vi "data_analysis main_correct.vi"() -> ()   [LabVIEW 2017]
uses:
  <vilib>/Analysis/baseanly.llb/Mean (DBL).vi
  <vilib>/Waveform/WDTFileIO.llb/Export Waveforms To Spreadsheet File (1D).vi
  <vilib>/Utility/file.llb/Read From Spreadsheet File (DBL).vi
  <vilib>/Analysis/NI_AALBase.lvlib
panel:
  in  "停止":bool
  out "Zmag trajectory":waveform(dbl) caption="元素"
  out "Ext.":dbl
  out "Z pos":waveform(dbl)(graph)
  out "Zmag pos":waveform(dbl)(graph)
  out "data name":string
  out "cursor pos":dbl
  out "cursor length":dbl
  out "zmag cursor pos":dbl
  out "zmag cursor length":dbl
  out "current bead":string
  in  "graphs":enum32{"raw data", "force calculation"}(tab)
  out "XY图":cluster{dbl[], dbl[]}(graph)
  in  "ref NO.":i32 min=0
  in  "remove drift":bool
  in  "sample rate":dbl=100.0
  in  "zero point offset":bool
  out "x_0":dbl caption="X0" format="%0.2f"
  out "y_0":dbl caption="Y0" format="%0.2f"
  out "z_0":dbl caption="Z0" format="%0.2f"
  in  "file save path":path
  in  "数据另存为":bool
  in  "data type":enum16{"tdms", "gr", "excel"}(ring)
  out "保存完成？":bool
  in  "file path":path
  in  "load data":bool
  in  "data info":i32(listbox)
  in  "bead NO.":i32 min=0
  in  "trajectory":i32 min=0
  out "Z mag":dbl
  in  "zmag or force":enum32{"zmag", "force"}(radio)
  in  "load excel":bool
  in  "B":dbl=-1.523
  in  "A":dbl=32.36
  in  "cali source":enum32{"X", "Y"}(radio)
  out "Power spectrum (um^2/Hz)":cluster{dbl[], "Spectrum out":dbl[]}[](graph)
  in  "Z_shift":dbl
  out "Force graph":cluster{dbl[], dbl[]}(graph)
  in  "accept":bool
  in  "force estimate":bool
  in  "Fit settings":T1={"#PSD Averages"=40, "Correct camera acquisition artifacts"=TRUE, "Autorange"=TRUE, "fstart (Hz)"=0.0, "Pendulum geometry"=FALSE, "Fit model"=FALSE} {"#PSD Averages" min=1}
  in  "fsampling (Hz)":dbl=2800.0
  in  "DNA length (um)":dbl=0.658
  out "Fit Results":T2
  out "fit data":dbl[][](array[numeric])
  in  "C":dbl
  in  "D":dbl
  # "load force-zmag"
  # "F="
  # "exp(                *Zmag)"
  # "*"
  # "exp(                *Zmag)"
  # "+"
  # "*"
  # "Fit parameters"
  # "Calculated quantities"
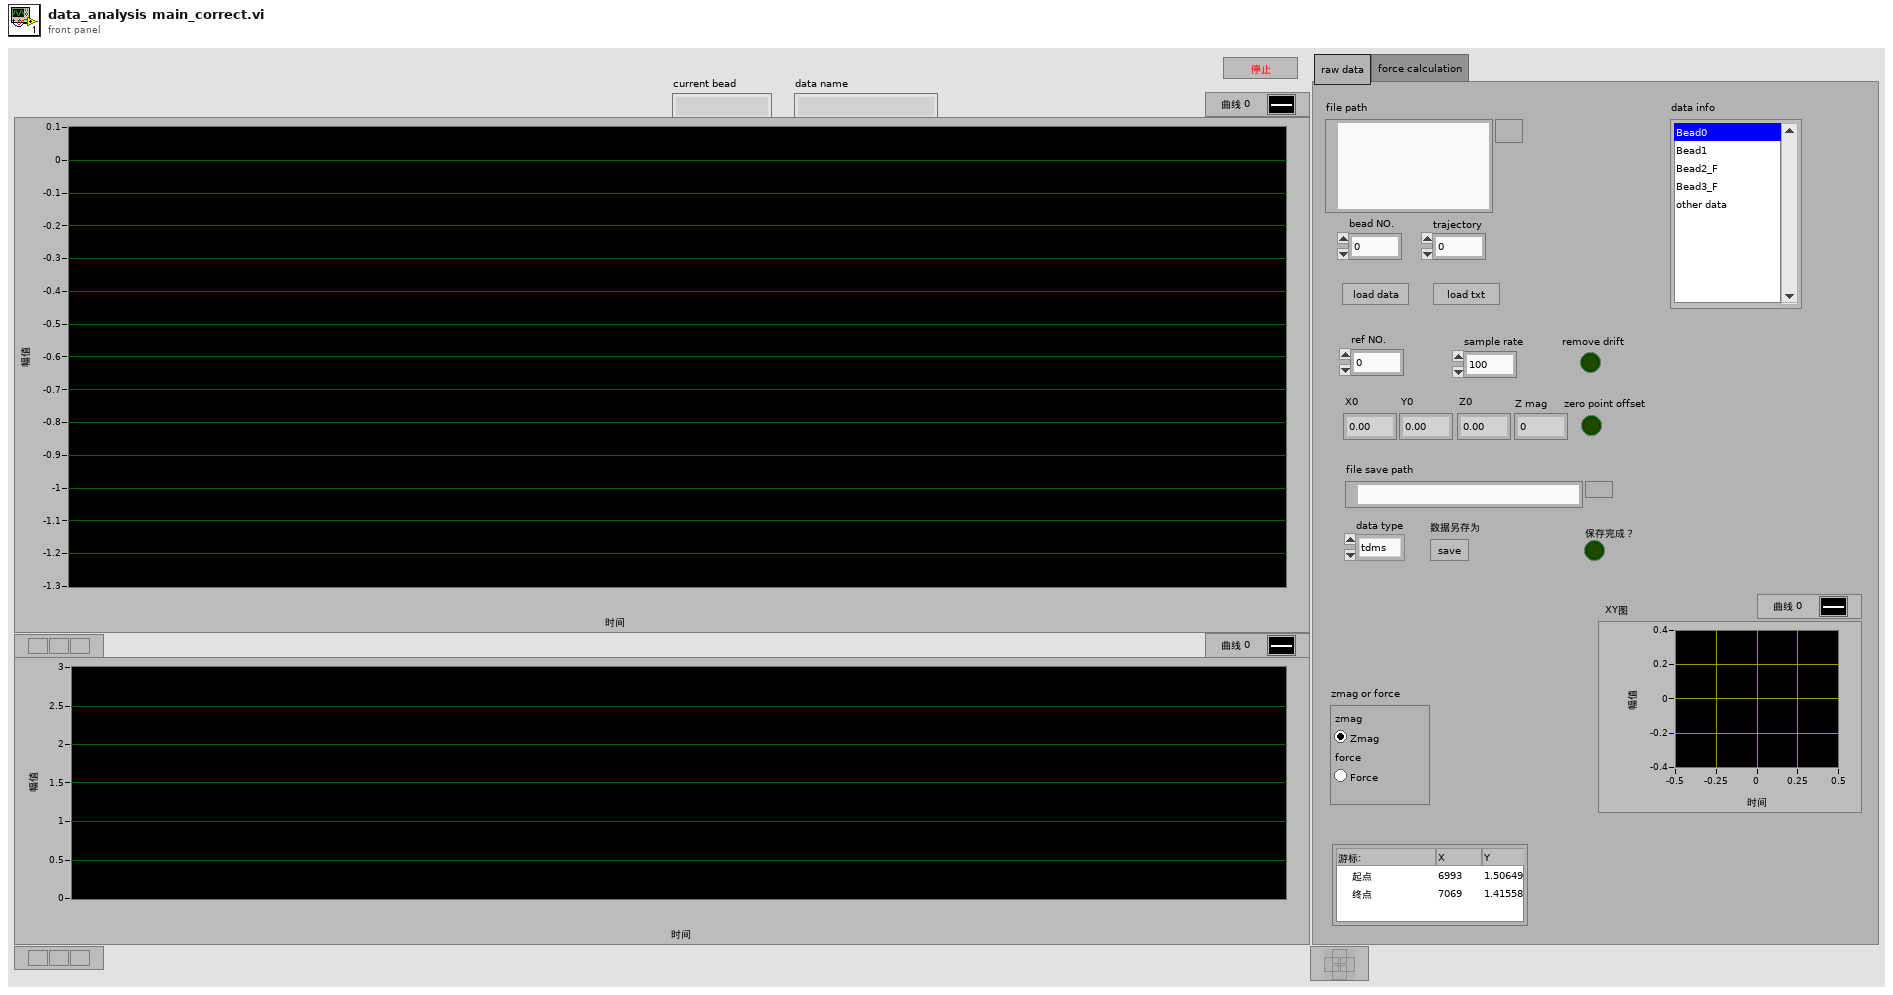
[diagram p1: front panel]
types:
  T1 = cluster{"#PSD Averages":u8, "Correct camera acquisition artifacts":bool, "Autorange":bool, "fstart (Hz)":dbl, "Pendulum geometry":bool, "Fit model":bool}
  T2 = cluster{"fcut (Hz)":dbl, "x2 (µm^2)":dbl, "Force (pN)":dbl, "Radius (µm)":dbl, "Apparent hydrodyn. radius (µm)":dbl, "fcut Error (Hz)":dbl, "x2 Error (µm^2)":dbl, "Force Error (pN)":dbl, "Radius Error (µm)":dbl, "Residue (unbiased)":dbl, "In range?":bool}
  T3 = enum16{"open", "open or create", "create or replace", "create", "open (read-only)"}
  T4 = enum16{"big-endian, network order", "native, host order", "little-endian"}
  T5 = enum16{"open", "replace", "create", "open or create", "replace or create", "replace or create with confirmation"}
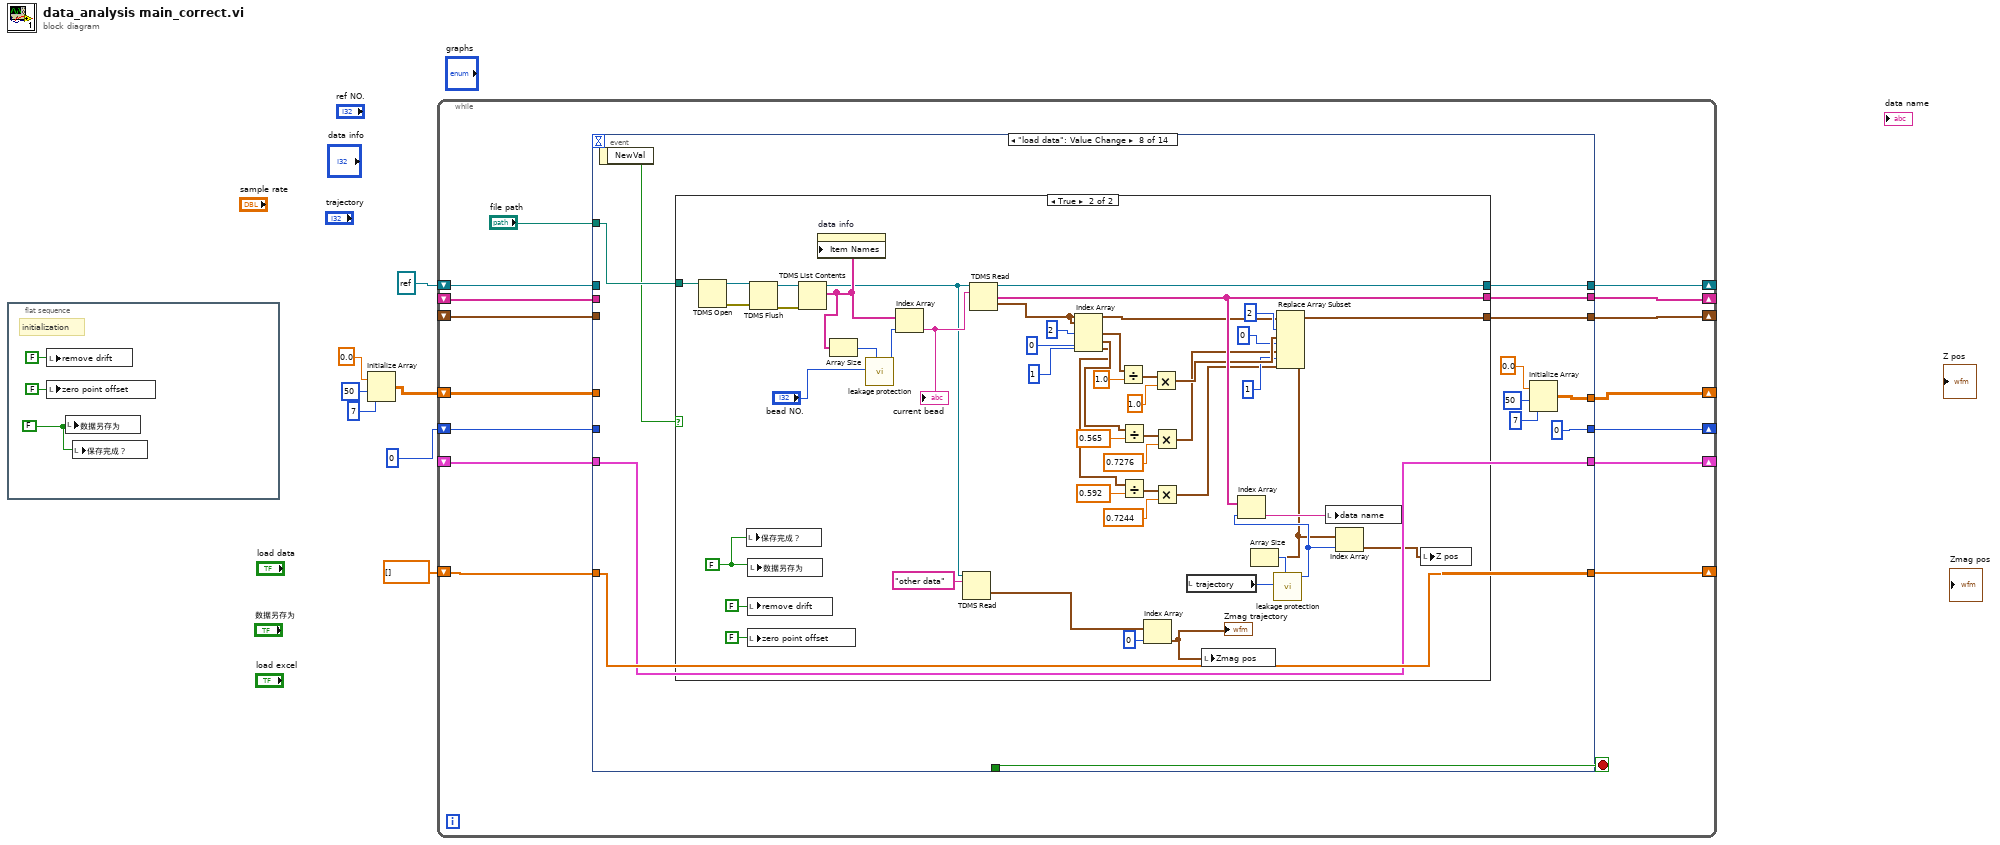
[diagram p0: block diagram]
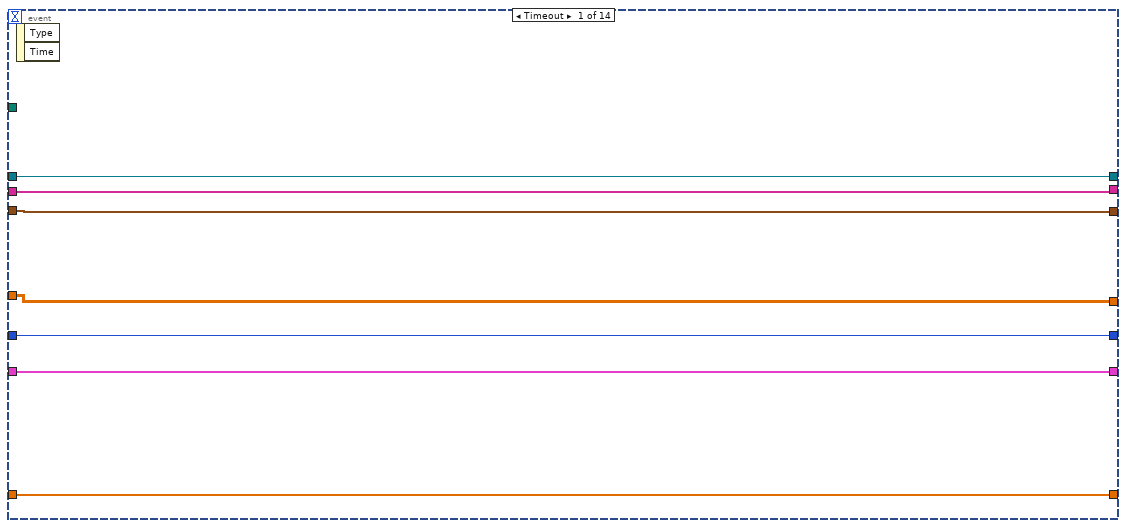
[diagram p2: hidden frame]
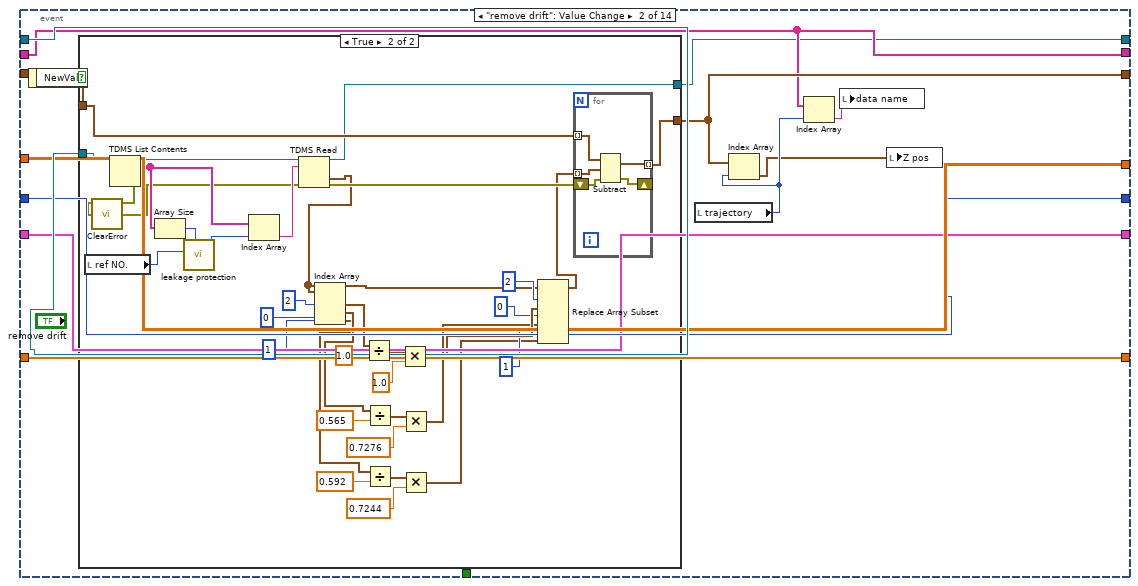
[diagram p3: hidden frame]
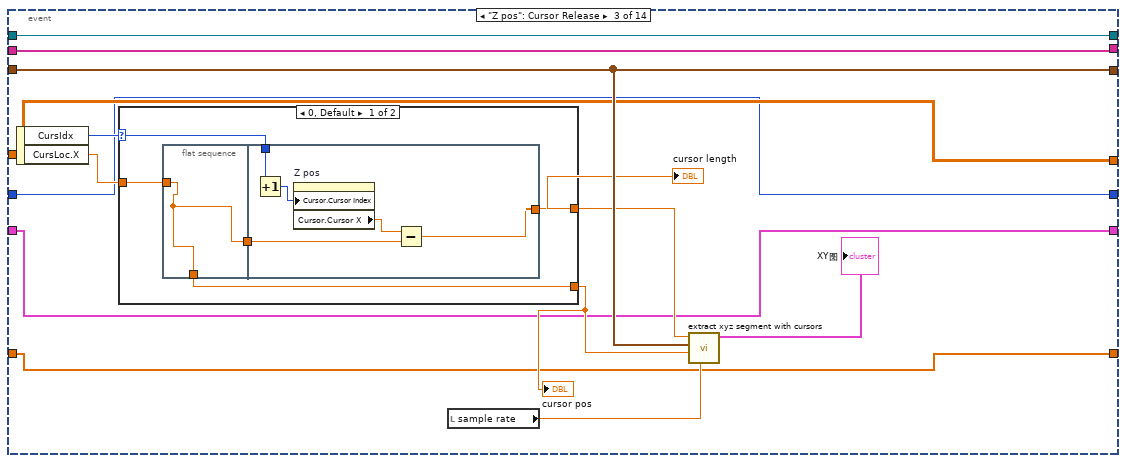
[diagram p5: hidden frame]
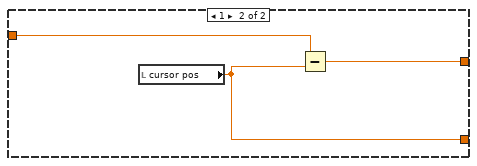
[diagram p6: hidden frame]
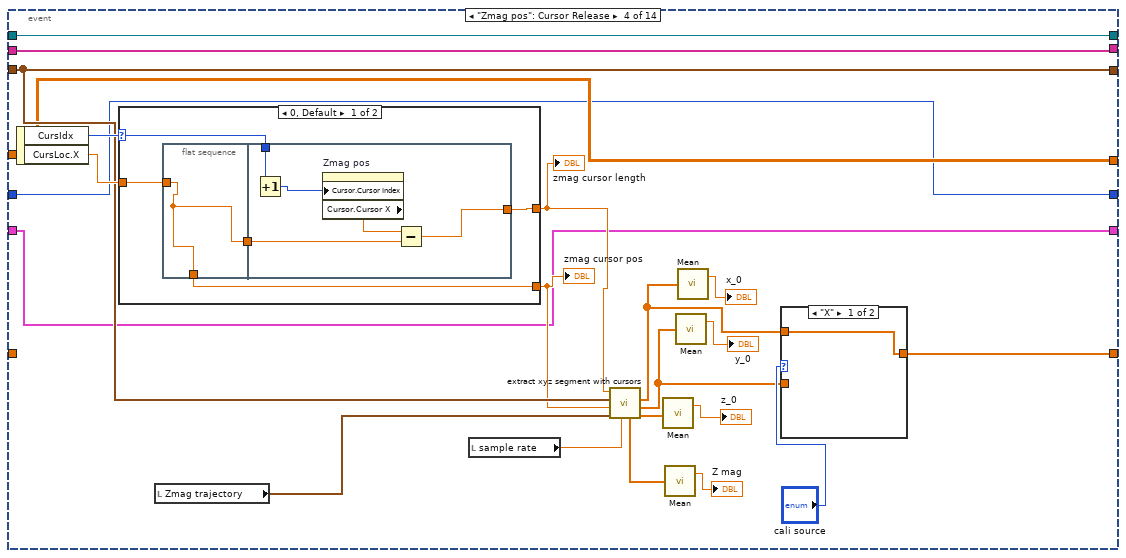
[diagram p7: hidden frame]
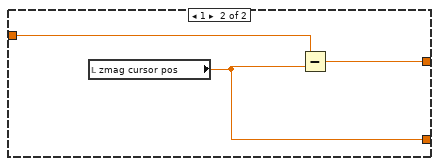
[diagram p9: hidden frame]
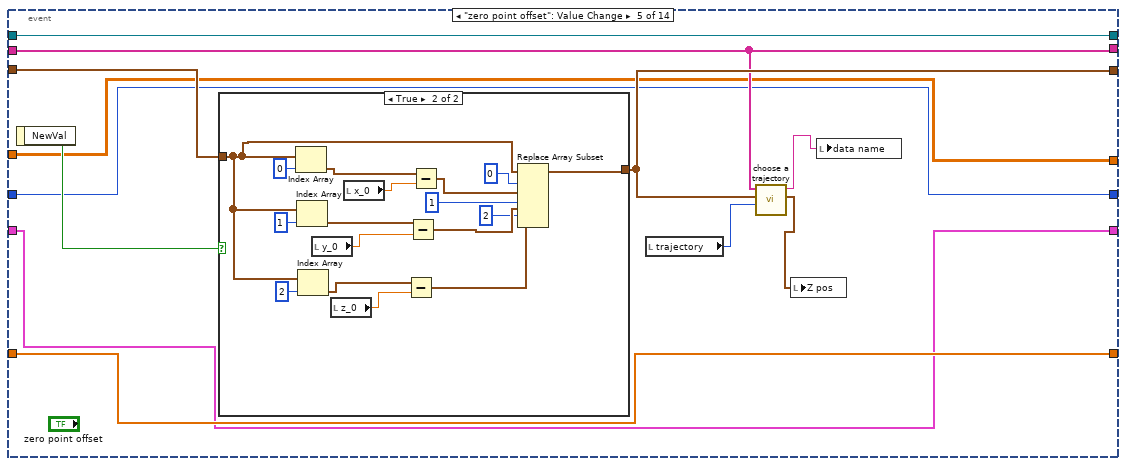
[diagram p10: hidden frame]
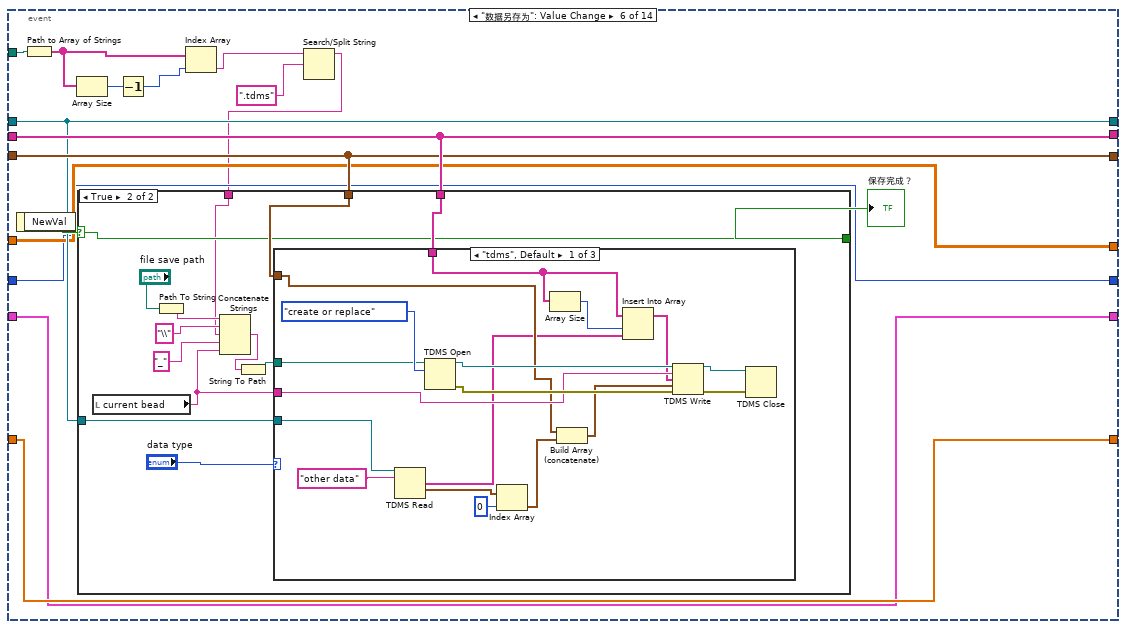
[diagram p12: hidden frame]
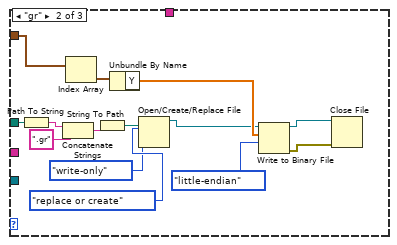
[diagram p14: hidden frame]
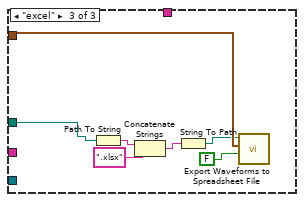
[diagram p15: hidden frame]
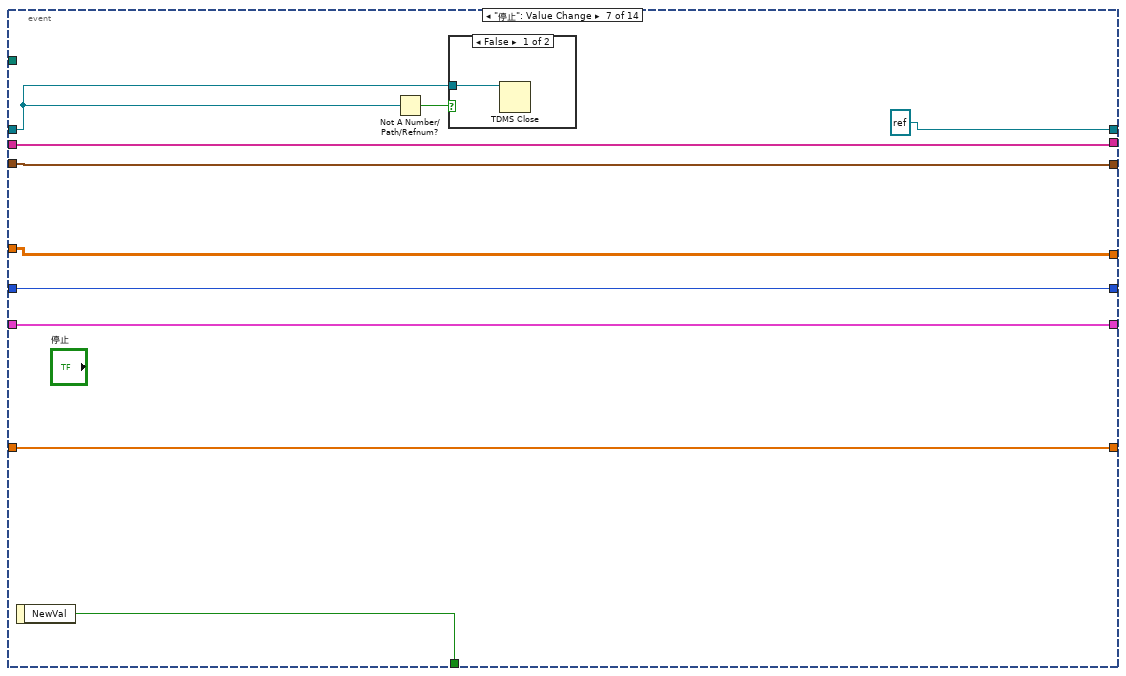
[diagram p16: hidden frame]
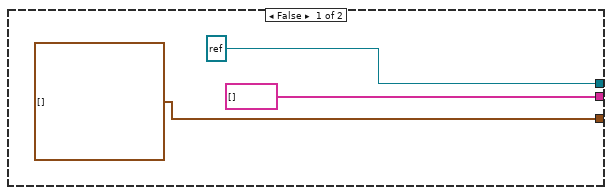
[diagram p18: hidden frame]
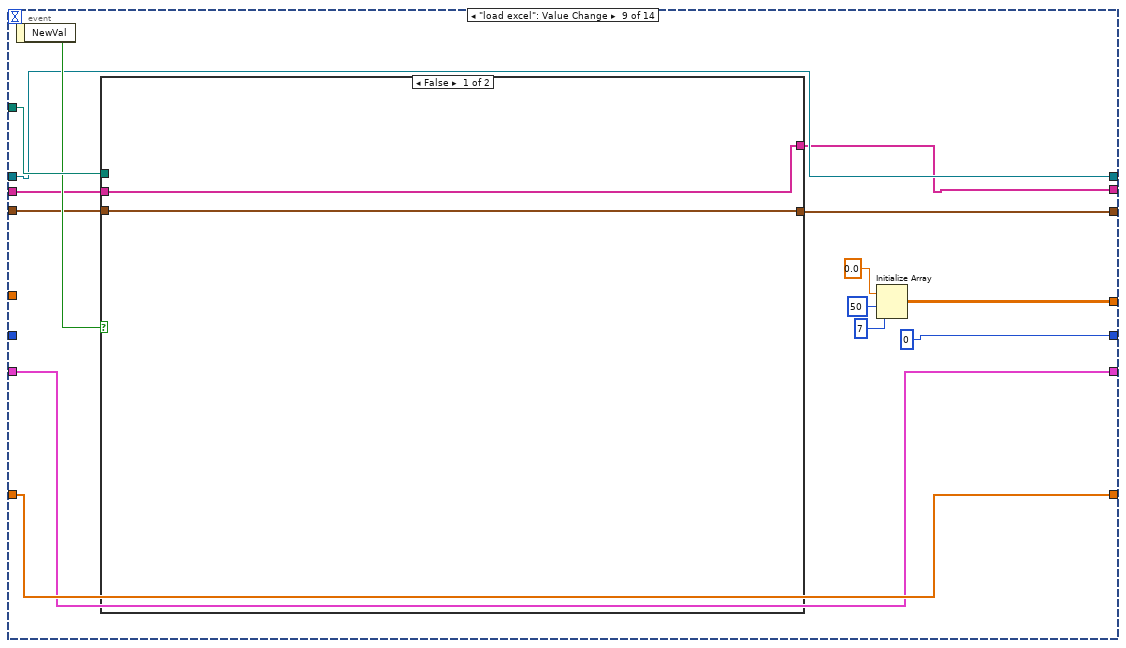
[diagram p19: hidden frame]
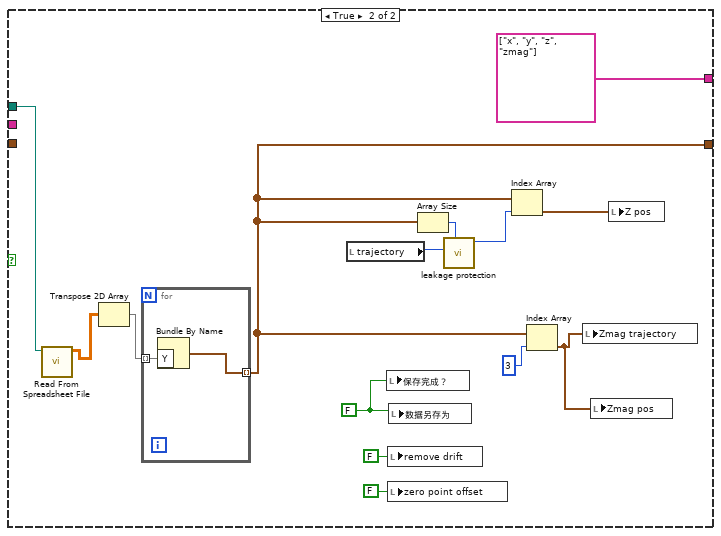
[diagram p20: hidden frame]
diagram:
  n1 = flat-sequence {
    frame #0 {
      w8 = FALSE ("数据另存为")
      # "initialization"
      n2 = local write "remove drift"(FALSE ("remove drift")) -> ()
      n3 = local write "zero point offset"(FALSE ("zero point offset")) -> ()
      n4 = local write "数据另存为"(w8) -> ()
      n5 = local write "保存完成？"(w8) -> ()
    }
  }
  n6 = Initialize Array(0.0 ("元素"), 50 ("维数大小"), 7 ("维数大小")) -> (w4:dbl[][])
  n7 = while {
    shift-right: [w24] -> _
    shift-left: refnum<k34> refnum ("tdms file out") -> [w19]
    shift-right: [w23] -> _
    shift-left: _ -> [w21]
    shift-right: [w22] -> _
    shift-left: _ -> [w20]
    shift-right: [w18] -> _
    shift-left: dbl[] [] ("Y") -> [w17]
    shift-right: [w16] -> _
    shift-left: _ -> [w15]
    shift-right: [w12] -> _
    shift-left: w4 -> [w14]
    shift-right: [w11] -> _
    shift-left: 0 -> [w13]
    stop <- w26 stop-if-true
    n8 = event "事件结构" shown="[7] \"load data\": Value Change" {
      selector: _ -> [_ _ _ _ _ _ _ _ _ _ _ _ _ _]
      dyn-events: _ -> [_ _ _ _ _ _ _ _ _ _ _ _ _ _]
      timeout: _ -> [_ _ _ _ _ _ _ _ _ _ _ _ _ _]
      tunnel: [_ _ _ _ _ _ w263 _ _ _ _ _ _ _] -> w26
      tunnel: "file path" -> [_ _ _ _ _ w191 _ w276 w341 _ _ _ _ _]
      tunnel: [w31 w40 w94 w127 w159 w196 refnum<k34> refnum ("tdms file out") w275 w332 w375 w385 w419 refnum<k34> refnum ("tdms file out") w465] -> w24
      tunnel: [w33 w42 w102 w138 w162 w199 w262 w274 w329 w374 w384 w418 w457 w466] -> w23
      tunnel: [w32 w43 w99 w135 w163 w198 w261 w273 w331 w373 w383 w417 w456 w468] -> w22
      tunnel: w21 -> [w33 w42 w102 w138 w162 w199 w262 _ w328 w374 w384 w418 w457 w466]
      tunnel: w20 -> [w32 w44 w99 w135 w165 w198 w261 _ w330 w373 w383 w417 w456 w468]
      tunnel: w19 -> [w31 w45 w94 w127 w159 w196 w255 _ w332 w375 w385 w419 w449 w465]
      tunnel: [w29 w37 w92 w118 w157 w194 w259 w271 w339 w372 w382 w401 w453 w461] -> w18
      tunnel: w17 -> [w29 w37 w92 _ w157 w194 w259 w271 w339 w372 w382 w401 w453 w461]
      tunnel: [w27 w35 w90 w124 w155 w192 w257 w270 w338 w369 w381 w415 w451 w459] -> w16
      tunnel: w15 -> [w27 w35 w90 w124 w155 w192 w257 w270 w338 _ w381 w415 w451 w459]
      tunnel: w14 -> [w30 w38 w93 w126 w158 w195 w260 _ _ w361 w380 w414 w454 w462]
      tunnel: w13 -> [w28 w36 w91 w125 w156 w193 w258 _ _ w360 w379 w413 w452 w460]
      tunnel: [w30 w38 w93 w126 w158 w195 w260 w266 w334 w361 w380 w407 w454 w462] -> w12
      tunnel: [w28 w36 w91 w125 w156 w193 w258 0 0 w360 w379 w404 w452 w460] -> w11
      event Timeout {
        n9 = event-data() -> ()  [unwired: 1 in, 2 out]
      }
      event "remove drift": Value Change {
        n10 = event-data() -> ("NewVal"=w46:bool)  [unwired: 1 in]
        n11 = case shown="True" w46 {
          tunnel: w45 -> [w47 w79]
          tunnel: w44 -> [w48 w76]
          tunnel: [w48 w74] -> w43
          tunnel: [w47 w73] -> w40
          frame False {
          }
          frame True {
            n12 = local read "ref NO."() -> (w78:i32)
            n13 = TDMS List Contents(7:w79) -> (0:w72:errorcluster, 2:w82:string[], 3:w84:refnum<k34>)  [unwired: 2 in, 1 out]
            n14 = call <vilib>:"ClearError.vi"("error in (no error)"=w72) -> ("error out"=w77:errorcluster)
            n15 = Array Size(array=w82) -> (size(s)=w81:i32)
            n16 = call "leakage protection.vi"("matrix size"=w81, "index in"=w78) -> ("index out"=w80:i32)  [unwired: 9 in]
            n17 = Index Array(array=w82, index=w80) -> (element=w83:string)
            n18 = TDMS Read(0:w84, 5:w83, 11:w77) -> (4:w73:refnum<k34>, 10:w50:waveform(dbl)[], 15:w75:errorcluster)  [unwired: 5 in, 3 out]
            n19 = Index Array(array=w50, index #1=2 ("索引"), index #2=0 ("index"), index #3=1 ("index")) -> (element #1=w66:waveform(dbl), element #2=w58:waveform(dbl), element #3=w53:waveform(dbl))
            n20 = Divide(x=w66, y=1.0) -> (x/y=w70:waveform(dbl))
            n21 = Divide(x=w58, y=0.565) -> (x/y=w60:waveform(dbl))
            n22 = Divide(x=w53, y=0.592) -> (x/y=w55:waveform(dbl))
            n23 = Multiply(x=w70, y=1.0) -> (x*y=w65:waveform(dbl))
            n24 = Multiply(x=w60, y=0.7276) -> (x*y=w57:waveform(dbl))
            n25 = Multiply(x=w55, y=0.7244) -> (x*y=w51:waveform(dbl))
            n26 = Replace Array Subset(array=w50, new element #1=w65, index #1=2 ("索引"), new element #2=w57, index #2=0 ("index"), new element #3=w51, index #3=1 ("index")) -> (w49:waveform(dbl)[])
            n27 = for {
              tunnel: w76 -> [w89] mode=indexing
              tunnel: w49 -> [w88] mode=indexing
              shift-right: [w86] -> _
              shift-left: w75 -> [w87]
              tunnel: [w85] -> w74 mode=indexing
              n28 = Subtract(1:w88, 2:w89, 4:w87) -> (0:w85:waveform(dbl), 3:w86:errorcluster)
            }
          }
        }
        n29 = local read "trajectory"() -> (w41:i32)
        n30 = Index Array(array=w43, index=w41) -> (element=w34:waveform(dbl))
        n31 = Index Array(array=w42, index=w41) -> (element=w39:string)
        n32 = local write "data name"(w39) -> ()
        n33 = local write "Z pos"(w34) -> ()
      }
      event "Z pos": Cursor Release {
        n34 = event-data() -> ("CursIdx"=w101:i32, "CursLoc.X"=w100:dbl)  [unwired: 1 in]
        n35 = case shown="0, Default" w101 {
          selector: w101 -> [w106 _]
          tunnel: w100 -> [w107 w116]
          tunnel: [w104 w115] -> w97
          tunnel: [w103 w114] -> w98
          frame 0, Default {
            n36 = flat-sequence {
              tunnel: w107 -> [w108]
              tunnel: [w108] -> w105
              tunnel: [w108] -> w103
              tunnel: w106 -> [w112]
              tunnel: w105 -> [w110]
              tunnel: [w109] -> w104
              frame #0 {
              }
              frame #1 {
                n37 = Increment(x=w112) -> (x+1=w113:i32)
                n38 = property on="Z pos" class="WFGraph (strict)"("Cursor.Cursor Index"=w113) -> ("Cursor.Cursor X"=w111:dbl)  [unwired: 2 in, 2 out]
                n39 = Subtract(x=w111, y=w110) -> (x-y=w109:dbl)
              }
            }
          }
          frame 1 {
            n40 = local read "cursor pos"() -> (w114:dbl)
            n41 = Subtract(x=w116, y=w114) -> (x-y=w115:dbl)
          }
        }
        "cursor length" <- w97
        "cursor pos" <- w98
        n42 = local read "sample rate"() -> (w96:dbl)
        n43 = call "extract xyz segment with cursors.vi"("sample rate"=w96, "cursor pos"=w98, "data"=w99, "cursor length"=w97) -> ("xy cluster"=→"XY图":cluster{dbl[], dbl[]})  [unwired: 3 in, 4 out]
      }
      event "Zmag pos": Cursor Release {
        n44 = event-data() -> ("CursIdx"=w137:i32, "CursLoc.X"=w136:dbl)  [unwired: 1 in]
        n45 = case shown="0, Default" w137 {
          selector: w137 -> [w144 _]
          tunnel: w136 -> [w145 w154]
          tunnel: [w142 w153] -> w133
          tunnel: [w141 w152] -> w134
          frame 0, Default {
            n46 = flat-sequence {
              tunnel: w145 -> [w146]
              tunnel: [w146] -> w143
              tunnel: [w146] -> w141
              tunnel: w144 -> [w151]
              tunnel: w143 -> [w150]
              tunnel: [w149] -> w142
              frame #0 {
              }
              frame #1 {
                n47 = Increment(x=w151) -> (x+1=w147:i32)
                n48 = property on="Zmag pos" class="WFGraph (strict)"("Cursor.Cursor Index"=w147) -> ("Cursor.Cursor X"=w148:dbl)  [unwired: 2 in, 2 out]
                n49 = Subtract(x=w148, y=w150) -> (x-y=w149:dbl)
              }
            }
          }
          frame 1 {
            n50 = local read "zmag cursor pos"() -> (w152:dbl)
            n51 = Subtract(x=w154, y=w152) -> (x-y=w153:dbl)
          }
        }
        "zmag cursor length" <- w133
        "zmag cursor pos" <- w134
        n52 = local read "Zmag trajectory"() -> (w123:waveform(dbl))
        n53 = local read "sample rate"() -> (w132:dbl)
        n54 = call "extract xyz segment with cursors.vi"("sample rate"=w132, "Zmag trajectory"=w123, "cursor pos"=w134, "data"=w135, "cursor length"=w133) -> ("Z"=w131:dbl[], "Y"=w119:dbl[], "X"=w117:dbl[], "Z mag"=w122:dbl[])  [unwired: 2 in, 1 out]
        n55 = call-poly <vilib>:"Mean.vi"("X"=w131) -> ("mean"=→"z_0":dbl)  [unwired: 1 out]
        n56 = call-poly <vilib>:"Mean.vi"("X"=w122) -> ("mean"=→"Z mag":dbl)  [unwired: 1 out]
        n57 = call-poly <vilib>:"Mean.vi"("X"=w119) -> ("mean"=→"y_0":dbl)  [unwired: 1 out]
        n58 = call-poly <vilib>:"Mean.vi"("X"=w117) -> ("mean"=→"x_0":dbl)  [unwired: 1 out]
        n59 = case shown="\"X\"" "cali source" {
          tunnel: w119 -> [_ w140]
          tunnel: [w139 w140] -> w118
          tunnel: w117 -> [w139 _]
          frame "X" {
          }
          frame "Y", Default {
          }
        }
      }
      event "zero point offset": Value Change {
        n60 = event-data() -> ("NewVal"=w166:bool)  [unwired: 1 in]
        n61 = case shown="True" w166 {
          tunnel: w165 -> [w167 w173]
          tunnel: [w167 w168] -> w163
          frame False {
          }
          frame True {
            n62 = Index Array(array=w173, index=0 ("索引")) -> (element=w181:waveform(dbl))
            n63 = Index Array(array=w173, index=1 ("索引")) -> (element=w179:waveform(dbl))
            n64 = Index Array(array=w173, index=2 ("索引")) -> (element=w177:waveform(dbl))
            n65 = local read "y_0"() -> (w178:dbl)
            n66 = local read "z_0"() -> (w176:dbl)
            n67 = local read "x_0"() -> (w180:dbl)
            n68 = Subtract(x=w177, y=w176) -> (x-y=w169:waveform(dbl))
            n69 = Subtract(x=w179, y=w178) -> (x-y=w171:waveform(dbl))
            n70 = Subtract(x=w181, y=w180) -> (x-y=w174:waveform(dbl))
            n71 = Replace Array Subset(array=w173, new element #1=w174, index #1=0 ("索引"), new element #2=w171, index #2=1 ("索引"), new element #3=w169, index #3=2 ("索引")) -> (w168:waveform(dbl)[])
          }
        }
        n72 = local read "trajectory"() -> (w164:i32)
        n73 = call "choose a trajectory.vi"("trajectory"=w164, "data"=w163, "bead info"=w162) -> ("trajectory"=w161:waveform(dbl), "data name"=w160:string)  [unwired: 7 in]
        n74 = local write "Z pos"(w161) -> ()
        n75 = local write "data name"(w160) -> ()
      }
      event "数据另存为": Value Change {
        n76 = event-data() -> ("NewVal"=w200:bool)  [unwired: 1 in]
        n77 = Path to Array of Strings(0:w191) -> (2:w190:string[])  [unwired: 1 out]
        n78 = Array Size(array=w190) -> (size(s)=w189:i32)
        n79 = Decrement(x=w189) -> (x-1=w188:i32)
        n80 = Index Array(array=w190, index=w188) -> (element=w187:string)
        n81 = Search/Split String(string=w187, search string/char (-)=".tdms" ("搜索字符串/字符(-)")) -> (substring before match=w185:string)  [unwired: 1 in, 2 out]
        n82 = case shown="True" w200 {
          selector: w200 -> [w201 w206]
          tunnel: w199 -> [_ w214]
          tunnel: w198 -> [_ w213]
          tunnel: [w201 w206] -> w197
          tunnel: w196 -> [_ w205]
          tunnel: w185 -> [_ w204]
          frame False {
          }
          frame True {
            n83 = local read "current bead"() -> (w202:string)
            n84 = Path To String(path="file save path") -> (string=w211:string)
            n85 = Concatenate Strings(w211, "\\" ("字符串"), w204, "_" ("字符串"), w202) -> (w209:string)
            n86 = String To Path(string=w209) -> (path=w208:path)
            n87 = case shown="\"tdms\", Default" "data type" {
              tunnel: w214 -> [w218 _ _]
              tunnel: w213 -> [w221 w240 w253]
              tunnel: w208 -> [w229 w242 w251]
              tunnel: w202 -> [w226 _ _]
              tunnel: w205 -> [w222 _ _]
              frame "tdms", Default {
                n88 = TDMS Read(0:w222, 5:"other data" ("组名称输入")) -> (8:w217:string[], 10:w224:waveform(dbl)[])  [unwired: 6 in, 4 out]
                n89 = TDMS Open(10:T3."create or replace" ("操作(0:open)"), 11:w229) -> (0:w230:errorcluster, 3:w231:refnum<k34>)  [unwired: 5 in]
                n90 = Index Array(array=w224, index=0 ("索引")) -> (element=w220:waveform(dbl))
                n91 = Array Size(array=w218) -> (size(s)=w215:i32)
                n92 = Build Array (concatenate)(w221, w220) -> (w219:waveform(dbl)[])
                n93 = Insert Into Array(array=w218, index=w215, new element=w217) -> (w216:string[])
                n94 = TDMS Write(0:w231, 5:w226, 7:w216, 9:w219, 11:w230) -> (4:w228:refnum<k34>, 15:w227:errorcluster)  [unwired: 1 in, 2 out]
                n95 = TDMS Close(8:w227, 11:w228) -> ()  [unwired: 2 out]
              }
              frame "gr" {
                n96 = Path To String(path=w242) -> (string=w245:string)
                n97 = Concatenate Strings(w245, ".gr" ("字符串")) -> (w243:string)
                n98 = Index Array(array=w240) -> (element=w239:waveform(dbl))  [unwired: 1 in]
                n99 = String To Path(string=w243) -> (path=w241:path)
                n100 = Unbundle By Name(w239) -> ("Y"=w237:dbl[])
                n101 = Open/Create/Replace File(file path (use dialog)=w241, operation (0:open)=T5."replace or create" ("操作(0:open)"), access (0:read/write)=enum16{"read/write", "read-only", "write-only"}."write-only" ("权限(0:read/write)")) -> (refnum out=w236:refnum<file>)  [unwired: 3 in, 2 out]
                n102 = Write to Binary File(file (use dialog)=w236, data=w237, 9:T4."little-endian" ("字节顺序(0:big-endian, network order)")) -> (refnum out=w235:refnum<file>, error out=w234:errorcluster)  [unwired: 3 in, 1 out]
                n103 = Close File(refnum=w235, error in=w234) -> ()  [unwired: 2 out]
              }
              frame "excel" {
                n104 = Path To String(path=w251) -> (string=w250:string)
                n105 = Concatenate Strings(w250, ".xlsx" ("字符串")) -> (w248:string)
                n106 = String To Path(string=w248) -> (path=w247:path)
                n107 = call-poly <vilib>:"Export Waveforms to Spreadsheet File.vi"("multiple time columns? (single:F)"=FALSE ("append to file? (new file:F)"), "waveforms"=w253, "file path (dialog if empty)"=w247) -> ()  [unwired: 7 in, 2 out]
              }
            }
          }
        }
        "保存完成？" <- w197
      }
      event "停止": Value Change {
        n108 = event-data() -> ("NewVal"=w263:bool)  [unwired: 1 in]
        n109 = Not A Number/Path/Refnum?(number/path/refnum=w255) -> (NaN/Path/Refnum?=w256:bool)
        n110 = case shown="False" w256 {
          tunnel: w255 -> [w264 _]
          frame False {
            n111 = TDMS Close(11:w264) -> ()  [unwired: 1 in, 2 out]
          }
          frame True {
          }
        }
      }
      event "load data": Value Change {
        n112 = event-data() -> ("NewVal"=w272:bool)  [unwired: 1 in]
        n113 = case shown="True" w272 {
          tunnel: w276 -> [_ w327]
          tunnel: [refnum<k34> refnum ("tdms file out") w325] -> w275
          tunnel: [string[] [] ("channel name(s) out") w324] -> w274
          tunnel: [waveform(dbl)[] [] ("data") w294] -> w273
          frame False {
          }
          frame True {
            w304 = FALSE ("数据另存为")
            n114 = TDMS Open(11:w327) -> (0:w315:errorcluster, 3:w316:refnum<k34>)  [unwired: 6 in]
            n115 = local write "保存完成？"(w304) -> ()
            n116 = local write "remove drift"(FALSE ("remove drift")) -> ()
            n117 = local write "zero point offset"(FALSE ("zero point offset")) -> ()
            n118 = local write "数据另存为"(w304) -> ()
            n119 = TDMS Flush(4:w315, 7:w316) -> (0:w314:errorcluster, 3:w313:refnum<k34>)
            n120 = TDMS List Contents(4:w314, 7:w313) -> (2:w321:string[], 3:w312:refnum<k34>)  [unwired: 1 in, 2 out]
            n121 = property on="data info" class="LstBox (strict)"("Item Names"=w321) -> ()  [unwired: 2 in, 2 out]
            n122 = Array Size(array=w321) -> (size(s)=w320:i32)
            n123 = call "leakage protection.vi"("matrix size"=w320, "index in"="bead NO.") -> ("index out"=w319:i32)  [unwired: 9 in]
            n124 = Index Array(array=w321, index=w319) -> (element=w326:string)
            "current bead" <- w326
            n125 = TDMS Read(0:w312, 5:"other data" ("组名称输入")) -> (10:w310:waveform(dbl)[])  [unwired: 6 in, 5 out]
            n126 = TDMS Read(0:w312, 5:w326) -> (4:w325:refnum<k34>, 8:w324:string[], 10:w298:waveform(dbl)[])  [unwired: 6 in, 3 out]
            n127 = Index Array(array=w298, index #1=2 ("索引"), index #2=0 ("index"), index #3=1 ("index")) -> (element #1=w296:waveform(dbl), element #2=w287:waveform(dbl), element #3=w282:waveform(dbl))
            n128 = Divide(x=w296, y=1.0) -> (x/y=w302:waveform(dbl))
            n129 = Divide(x=w287, y=0.565) -> (x/y=w289:waveform(dbl))
            n130 = Divide(x=w282, y=0.592) -> (x/y=w284:waveform(dbl))
            n131 = Index Array(array=w310, index=0 ("索引")) -> (element=w305:waveform(dbl))
            "Zmag trajectory" <- w305
            n132 = Multiply(x=w302, y=1.0) -> (x*y=w295:waveform(dbl))
            n133 = Multiply(x=w289, y=0.7276) -> (x*y=w286:waveform(dbl))
            n134 = Multiply(x=w284, y=0.7244) -> (x*y=w280:waveform(dbl))
            n135 = local read "trajectory"() -> (w318:i32)
            n136 = local write "Zmag pos"(w305) -> ()
            n137 = Replace Array Subset(array=w298, new element #1=w295, index #1=2 ("索引"), new element #2=w286, index #2=0 ("index"), new element #3=w280, index #3=1 ("index")) -> (w294:waveform(dbl)[])
            n138 = Array Size(array=w294) -> (size(s)=w322:i32)
            n139 = call "leakage protection.vi"("matrix size"=w322, "index in"=w318) -> ("index out"=w323:i32)  [unwired: 9 in]
            n140 = Index Array(array=w324, index=w323) -> (element=w317:string)
            n141 = local write "data name"(w317) -> ()
            n142 = Index Array(array=w294, index=w323) -> (element=w299:waveform(dbl))
            n143 = local write "Z pos"(w299) -> ()
          }
        }
        n144 = Initialize Array(0.0 ("元素"), 50 ("维数大小"), 7 ("维数大小")) -> (w266:dbl[][])
      }
      event "load excel": Value Change {
        n145 = event-data() -> ("NewVal"=w340:bool)  [unwired: 1 in]
        n146 = case shown="False" w340 {
          tunnel: w341 -> [_ w350]
          tunnel: [w343 w348] -> w331
          tunnel: w330 -> [w343 _]
          tunnel: [w342 string[] ["x", "y", "z", "zmag"] ("channel name(s) out")] -> w329
          tunnel: w328 -> [w342 _]
          frame False {
          }
          frame True {
            w351 = FALSE ("数据另存为")
            n147 = call-poly <vilib>:"Read From Spreadsheet File.vi"("file path (dialog if empty)"=w350) -> ("all rows"=w346:dbl[][])  [unwired: 6 in, 4 out]
            n148 = Transpose 2D Array(2D array=w346) -> (transposed array=w345:dbl[][])
            n149 = for {
              tunnel: w345 -> [w359] mode=indexing
              tunnel: [w358] -> w348 mode=indexing
              n150 = Bundle By Name("Y"=w359) -> (w358:waveform(dbl))  [unwired: 1 in]
            }
            n151 = local read "trajectory"() -> (w355:i32)
            n152 = local write "保存完成？"(w351) -> ()
            n153 = local write "remove drift"(FALSE ("remove drift")) -> ()
            n154 = local write "zero point offset"(FALSE ("zero point offset")) -> ()
            n155 = local write "数据另存为"(w351) -> ()
            n156 = Array Size(array=w348) -> (size(s)=w356:i32)
            n157 = call "leakage protection.vi"("matrix size"=w356, "index in"=w355) -> ("index out"=w357:i32)  [unwired: 9 in]
            n158 = Index Array(array=w348, index=w357) -> (element=w349:waveform(dbl))
            n159 = Index Array(array=w348, index=3 ("索引")) -> (element=w347:waveform(dbl))
            n160 = local write "Zmag trajectory"(w347) -> ()
            n161 = local write "Zmag pos"(w347) -> ()
            n162 = local write "Z pos"(w349) -> ()
          }
        }
        n163 = Initialize Array(0.0 ("元素"), 50 ("维数大小"), 7 ("维数大小")) -> (w334:dbl[][])
      }
      event "force estimate": Value Change {
        n164 = event-data() -> ()  [unwired: 1 in, 1 out]
        n165 = local read "z_0"() -> (w364:dbl)
        n166 = Subtract(x="DNA length (um)", y="Z_shift") -> (x-y=w365:dbl)
        n167 = Add(x=w365, y=w364) -> (x+y=w363:dbl)
        "Ext." <- w363
        n168 = call "PSD fitting.vi"("DNA length (µm)"=w363, "fsampling (Hz)"="fsampling (Hz)", "Fit settings"="Fit settings", "X/Y data"=w372) -> ("Fit Results"=w369:T2, "Power spectrum (um^2/Hz)"=→"Power spectrum (um^2/Hz)":cluster{dbl[], "Spectrum out":dbl[]}[])  [unwired: 6 in]
        "Fit Results" <- w369
        n169 = local write "accept"(FALSE ("accept")) -> ()
      }
      event "zmag or force": Value Change {
        n170 = event-data() -> ()  [unwired: 1 in, 1 out]
        n171 = local read "Zmag trajectory"() -> (w377:waveform(dbl))
        n172 = case shown="\"force\"" "zmag or force" {
          tunnel: w377 -> [w386 w395]
          tunnel: [w386 w396] -> w376
          frame "zmag", Default {
          }
          frame "force" {
            n173 = Unbundle By Name(w395) -> ("Y"=w390:dbl[])
            n174 = Multiply(x=w390, y="B") -> (x*y=w399:dbl[])
            n175 = Exponential(1:w399) -> (0:w398:dbl[])
            n176 = Multiply(x=w390, y="D") -> (x*y=w392:dbl[])
            n177 = Multiply(x=w398, y="A") -> (x*y=w388:dbl[])
            n178 = Exponential(1:w392) -> (0:w393:dbl[])
            n179 = Multiply(x=w393, y="C") -> (x*y=w389:dbl[])
            n180 = Add(x=w388, y=w389) -> (x+y=w387:dbl[])
            n181 = Bundle By Name(cluster=w395, "Y"=w387) -> (w396:waveform(dbl))
          }
        }
        n182 = local write "Zmag pos"(w376) -> ()
      }
      event "accept": Value Change {
        n183 = event-data() -> ()  [unwired: 1 in, 1 out]
        n184 = case shown="False" "accept" {
          tunnel: w415 -> [_ w446]
          tunnel: w414 -> [w420 w432]
          tunnel: w413 -> [w421 w424]
          tunnel: [w420 w422] -> w407
          tunnel: [w421 w434] -> w404
          frame False {
          }
          frame True {
            n185 = Unbundle By Name(w446) -> ("Force (pN)"=w445:dbl, "Force Error (pN)"=w440:dbl, "Radius (µm)"=w439:dbl, "Radius Error (µm)"=w438:dbl, "fcut (Hz)"=w425:dbl)
            n186 = local read "Z mag"() -> (w428:dbl)
            n187 = local read "Ext."() -> (w430:dbl)
            n188 = Replace Array Subset(array=w432, new element=w430, index (row)=w424, index (col)=0 ("禁用的索引 (列)")) -> (w431:dbl[][])
            n189 = Replace Array Subset(array=w431, new element=w445, index (row)=w424, index (col)=1 ("禁用的索引 (列)")) -> (w437:dbl[][])
            n190 = Replace Array Subset(array=w437, new element=w440, index (row)=w424, index (col)=2 ("禁用的索引 (列)")) -> (w436:dbl[][])
            n191 = Replace Array Subset(array=w436, new element=w439, index (row)=w424, index (col)=3 ("禁用的索引 (列)")) -> (w435:dbl[][])
            n192 = Replace Array Subset(array=w435, new element=w438, index (row)=w424, index (col)=4 ("禁用的索引 (列)")) -> (w427:dbl[][])
            n193 = Replace Array Subset(array=w427, new element=w428, index (row)=w424, index (col)=5 ("禁用的索引 (列)")) -> (w423:dbl[][])
            n194 = Replace Array Subset(array=w423, new element=w425, index (row)=w424, index (col)=6 ("禁用的索引 (列)")) -> (w422:dbl[][])
            n195 = Increment(x=w424) -> (x+1=w434:i32)
          }
        }
        n196 = Array Subset(array=w407, index (row)=0 ("索引"), length (row)=w404, index (col)=0 ("索引"), length (col)=7 ("长度")) -> (w402:dbl[][])
        "fit data" <- w402
        n197 = Index Array(array=w402, index (col) #1=0 ("禁用的索引 (列)"), index (col) #2=1 ("索引 (列)")) -> (element #1=w411:dbl[], element #2=w409:dbl[])  [unwired: 2 in]
        n198 = Bundle(w411, w409) -> (→"Force graph":cluster{dbl[], dbl[]})  [unwired: 1 in]
      }
      event "file path": Value Change {
        n199 = event-data() -> ("NewVal"=w455:path)  [unwired: 1 in, 4 out]
        n200 = local write "file path"(w455) -> ()
        n201 = local write "bead NO."(0 ("bead NO.")) -> ()
        n202 = Not A Number/Path/Refnum?(number/path/refnum=w449) -> (NaN/Path/Refnum?=w448:bool)
        n203 = case shown="False" w448 {
          tunnel: w449 -> [w458 _]
          frame False {
            n204 = TDMS Close(11:w458) -> ()  [unwired: 1 in, 2 out]
          }
          frame True {
          }
        }
      }
      event "trajectory": Value Change {
        n205 = event-data() -> ("NewVal"=w467:i32)  [unwired: 1 in]
        n206 = call "choose a trajectory.vi"("trajectory"=w467, "data"=w468, "bead info"=w466) -> ("trajectory"=w463:waveform(dbl), "data name"=w464:string)  [unwired: 7 in]
        n207 = local write "data name"(w464) -> ()
        n208 = local write "Z pos"(w463) -> ()
      }
    }
  }
